vi "Get - Object Origin.vi"(0 "reference in":refnum<class "Registration.lvclass">, 5 "error in (no error)":errorcluster) -> (13 "Object Origin":enum16{"New/Created", "Existing"}(ring), 14 "reference out":refnum<class "Registration.lvclass">, 19 "error out":errorcluster)   [LabVIEW 2022 SP3, in "Registration.lvclass"]
uses:
  Registration.lvclass
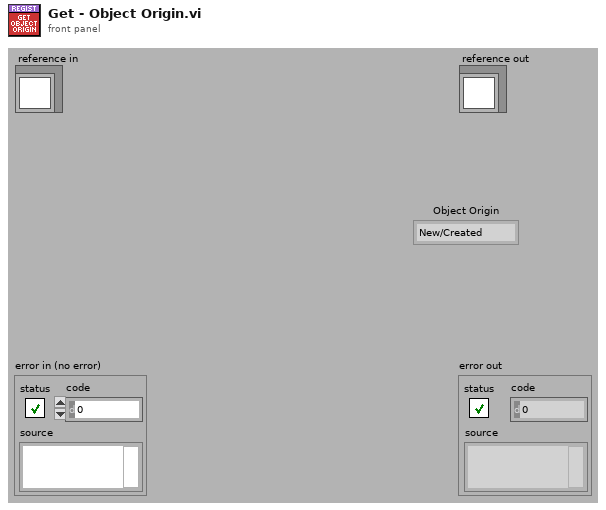
[diagram p1: front panel]
types:
  T1 = typedef "Registration.lvclass/ObjectAttributes.ctl" = cluster{"Registration Info":T2, "Object Origin":enum16{"New/Created", "Existing"}}
  T2 = typedef "Registration.lvclass/Registration Info.ctl" = cluster{"First Name":string, "Last Name":string, "Registration Code":string, "Registration Level":T3}
  T3 = typedef "Registration.lvclass/Registration Type.ctl" = enum16{"Unregistered", "Registered - Full Activation", "Not Required- Full Activation"}
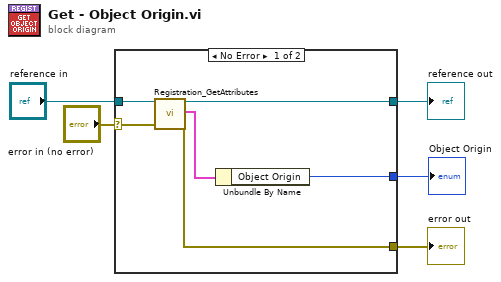
[diagram p0: block diagram]
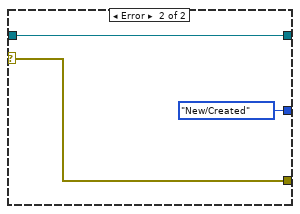
[diagram p2: hidden frame]
diagram:
  n1 = case shown="No Error" "error in (no error)" {
    selector: "error in (no error)" -> [w11 w14]
    tunnel: [w10 w14] -> w4
    tunnel: [w9 w13] -> w2
    tunnel: "reference in" -> [w7 w13]
    tunnel: [w6 enum16{"New/Created", "Existing"}."New/Created" ("Object Origin")] -> w1
    frame No Error {
      n2 = call "Registration_GetAttributes.vi"("reference in"=w7, "error in (no error)"=w11) -> ("reference out"=w9:refnum<class "Registration.lvclass">, "attributes"=w8:T1, "error out"=w10:errorcluster)  [unwired: 14 in, 1 out]
      n3 = Unbundle By Name(w8) -> ("Object Origin"=w6:enum16{"New/Created", "Existing"})
    }
    frame Error {
    }
  }
  "error out" <- w4
  "reference out" <- w2
  "Object Origin" <- w1
